vi "Read_Write_Temp_Cluster.vi"(3 "Template Info Array":T2[](array[typedef]) {"Tolerance" min=0.0 format="%#.4f"}, 4 "Mode":T1, 5 "Template File":path) -> (0 "Template Info Array Out":T2[](array[typedef]) {"Tolerance" min=0.0 format="%#.4f"})   [LabVIEW 2010]
uses:
  File_Template_Clus.ctl
  Controls/Global_mode.ctl
panel:
  # "> 20  or\n<20   or\n =20"
  # "<<Characters_to_Match>>  <<Replace_Whole_String_with_this>>"
  # "Channel_Name contains Characters to match or\nChannel_Name does not contain Characters to match"
  # "Channel_Name_A + Channel_Name_B or\nConcatenate Channel_Name_A and Channel_Name_B"
  # "> 20  or\n<20   or\n =20"
  # "<<Characters_to_Match>>  <<Replace_Whole_String_with_this>>"
  # "Channel_Name contains Characters to match or\nChannel_Name does not contain Characters to match"
  # "Channel_Name_A + Channel_Name_B or\nConcatenate Channel_Name_A and Channel_Name_B"
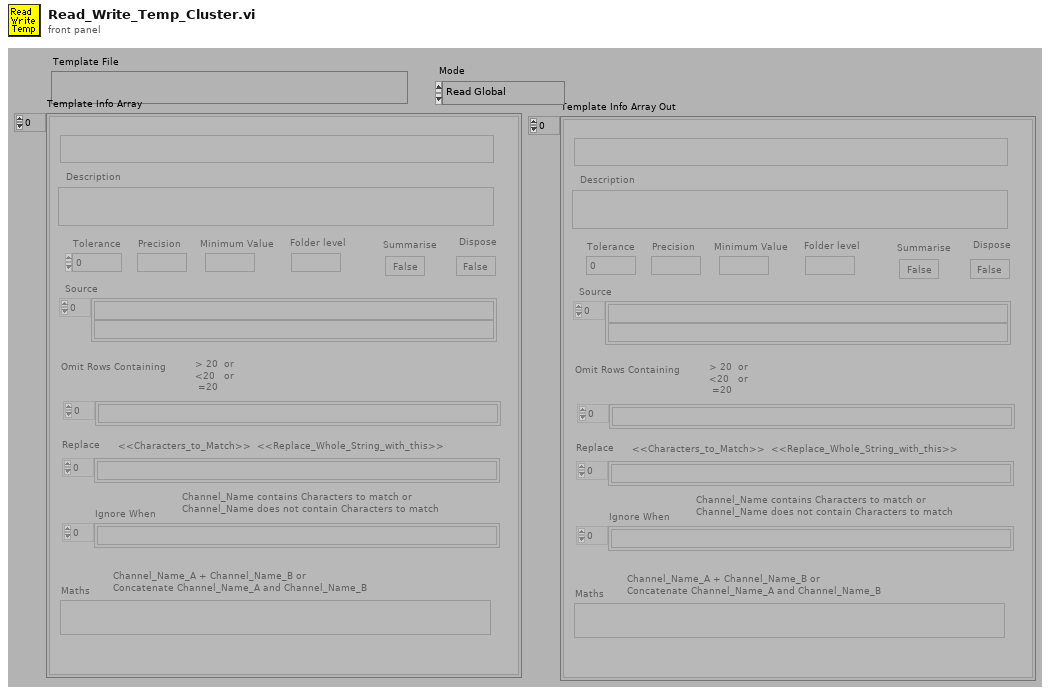
[diagram p1: front panel]
types:
  T1 = typedef "Global_mode.ctl" = enum16{"Read Global", "Load Global From File", "Write Global to File"}
  T2 = typedef "File_Template_Clus.ctl" = cluster{"Template Channel Name":string, "Description":string, "Tolerance":dbl, "Precision":string, "Folder level":string, "Source":string[], "Replace":string[], "Summarise":bool, "Dispose":bool, "Minimum Value":string, "Maths":string, "Omit Rows Containing":string[], "Ignore When":string[]}
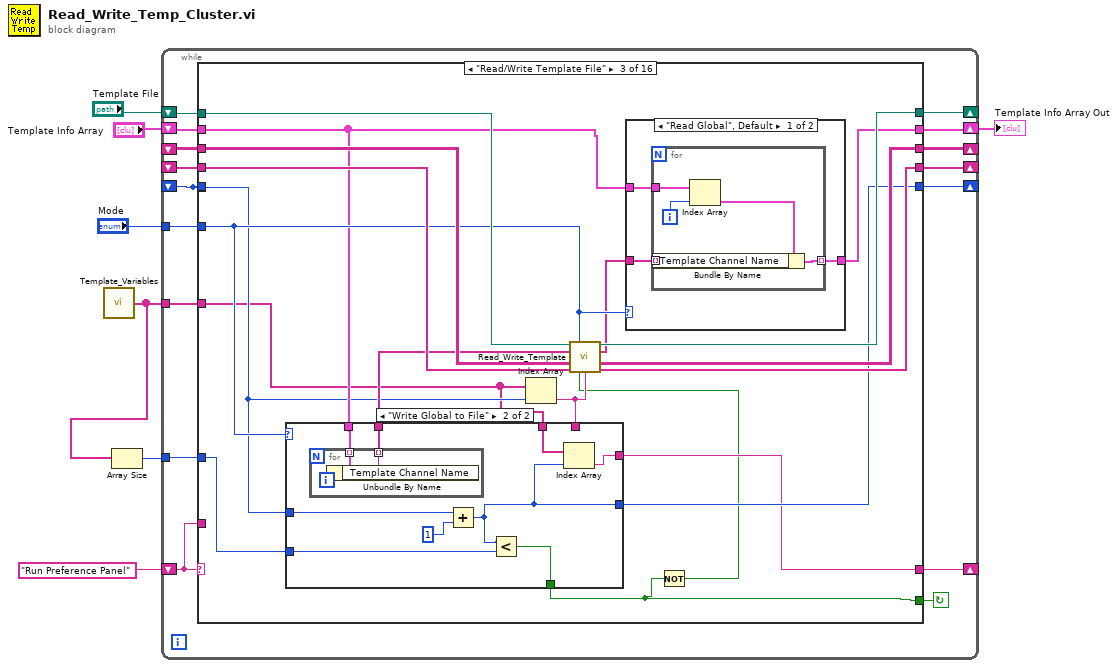
[diagram p0: block diagram]
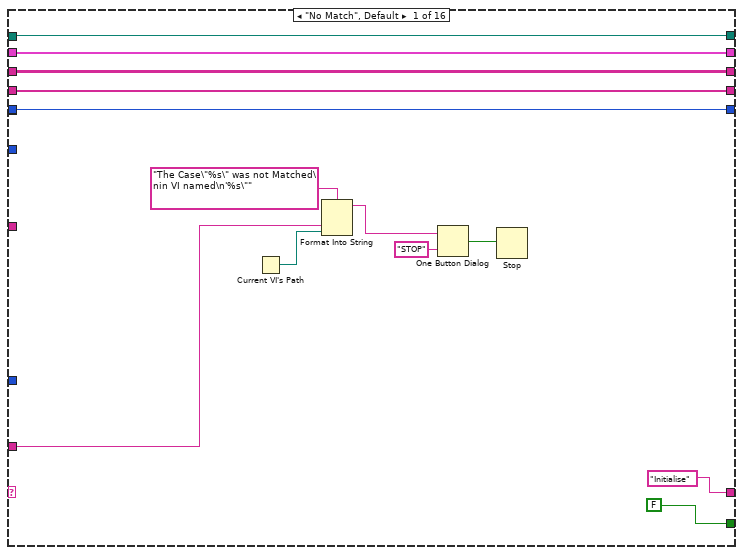
[diagram p2: hidden frame]
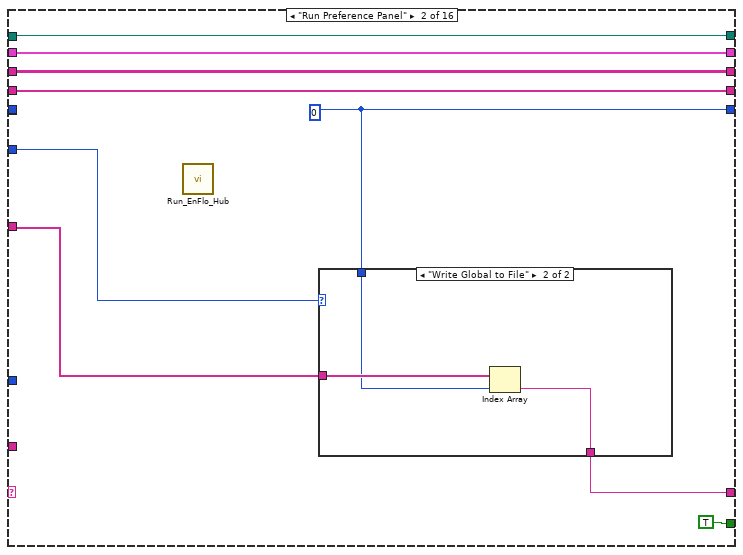
[diagram p3: hidden frame]
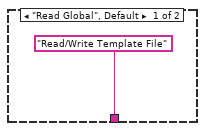
[diagram p4: hidden frame]
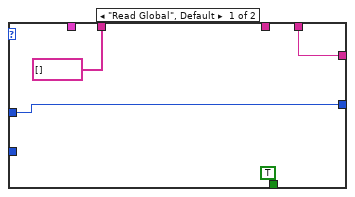
[diagram p6: hidden frame]
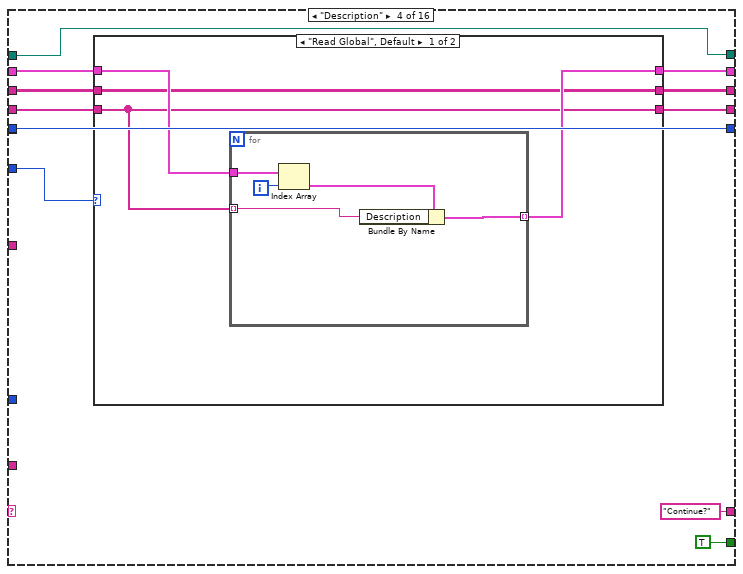
[diagram p7: hidden frame]
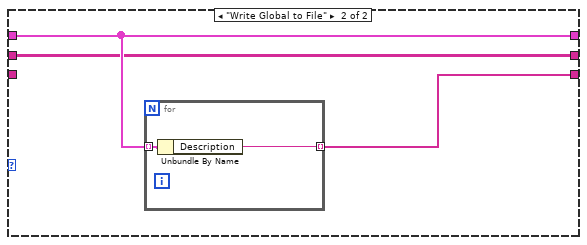
[diagram p8: hidden frame]
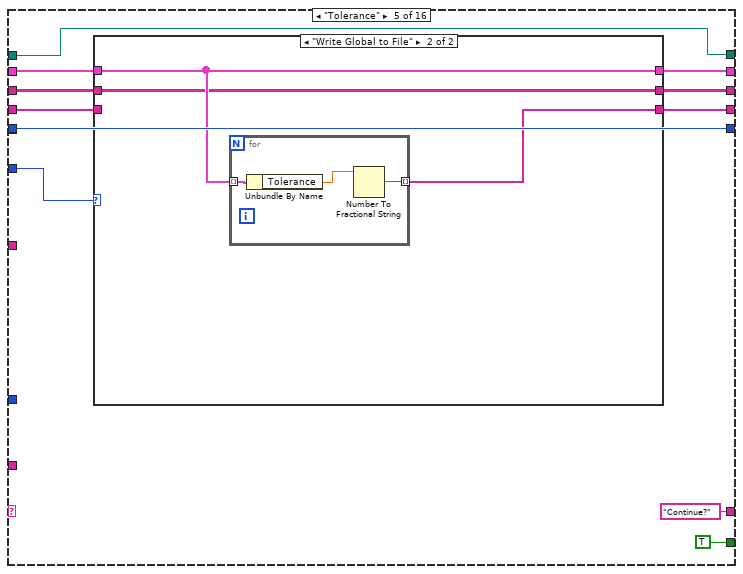
[diagram p9: hidden frame]
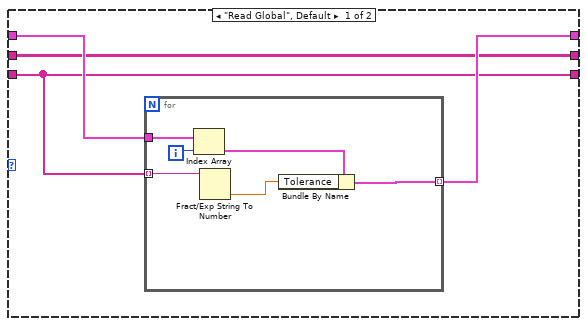
[diagram p10: hidden frame]
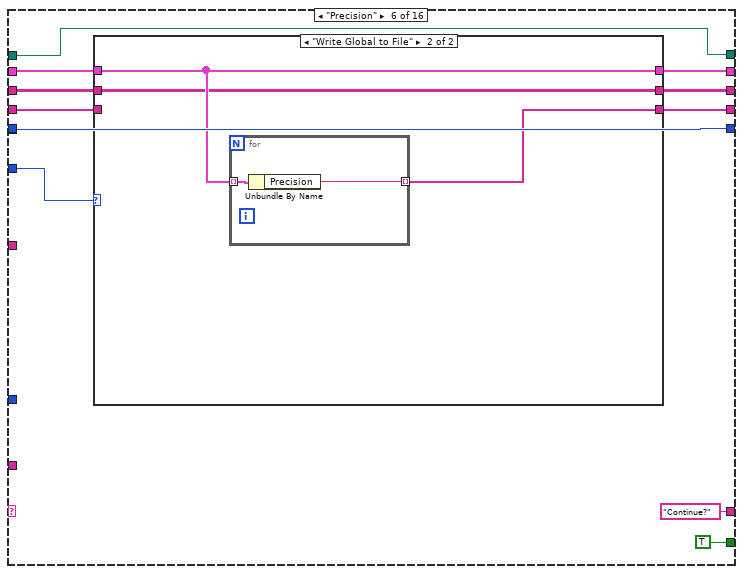
[diagram p11: hidden frame]
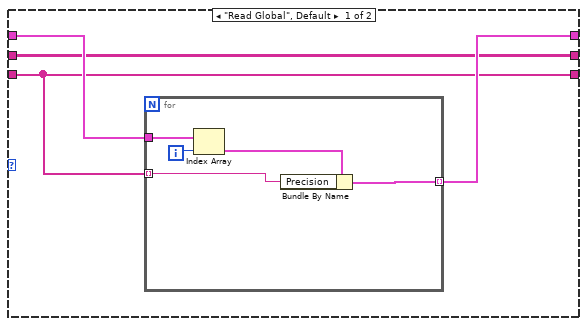
[diagram p12: hidden frame]
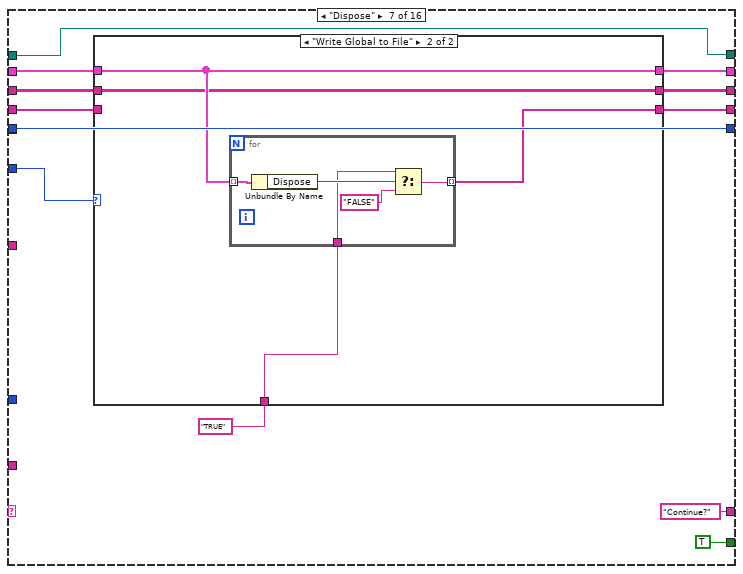
[diagram p13: hidden frame]
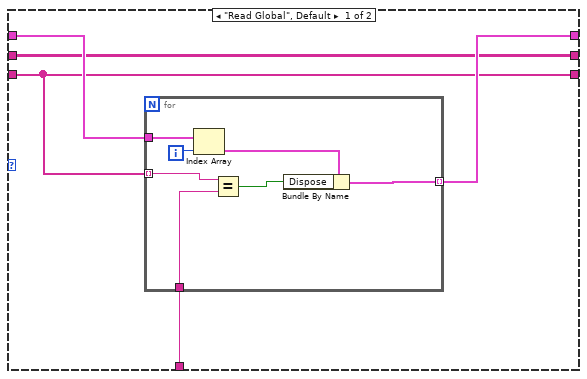
[diagram p14: hidden frame]
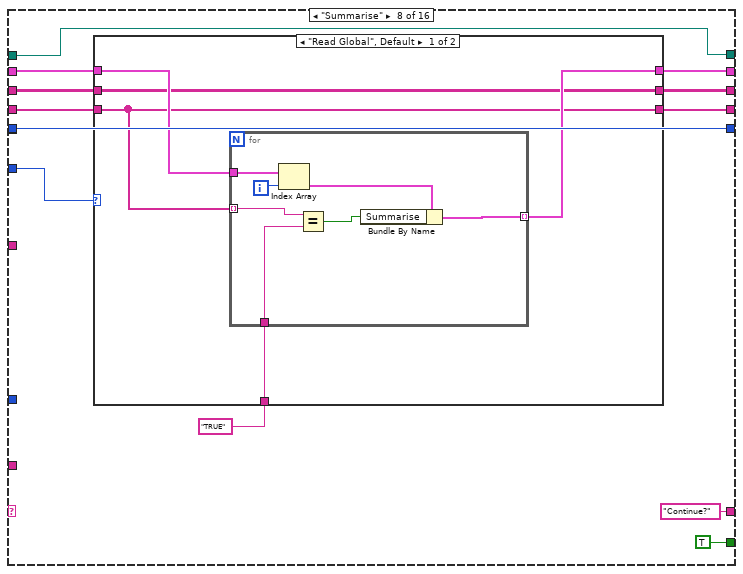
[diagram p15: hidden frame]
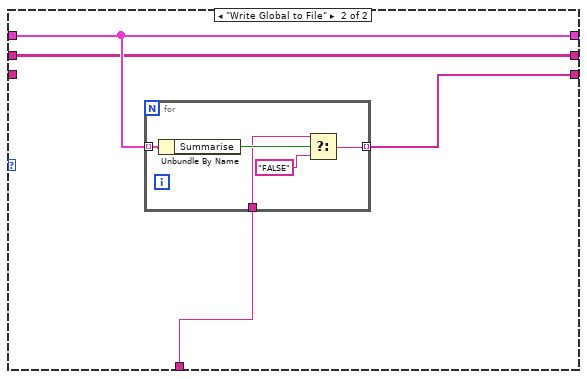
[diagram p16: hidden frame]
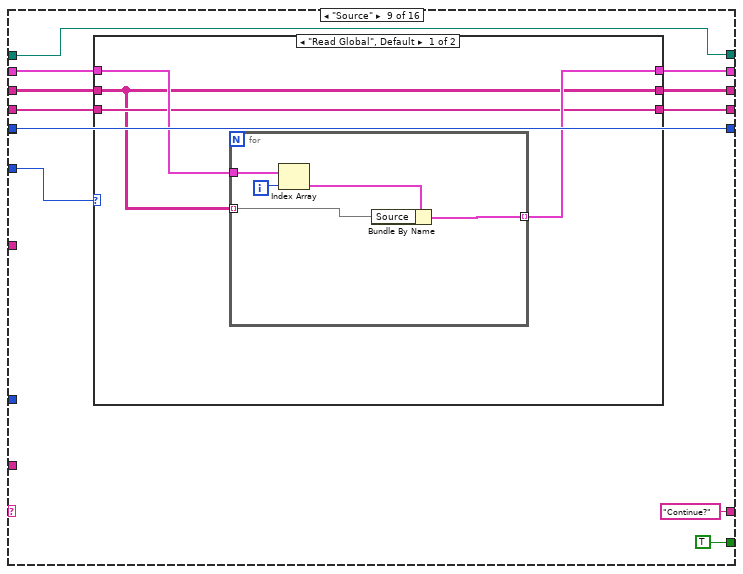
[diagram p17: hidden frame]
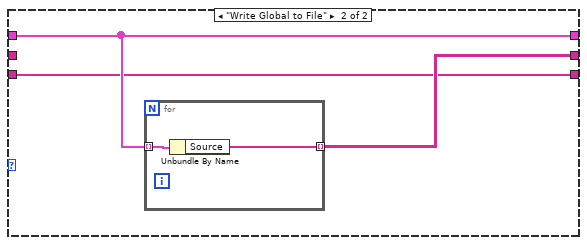
[diagram p18: hidden frame]
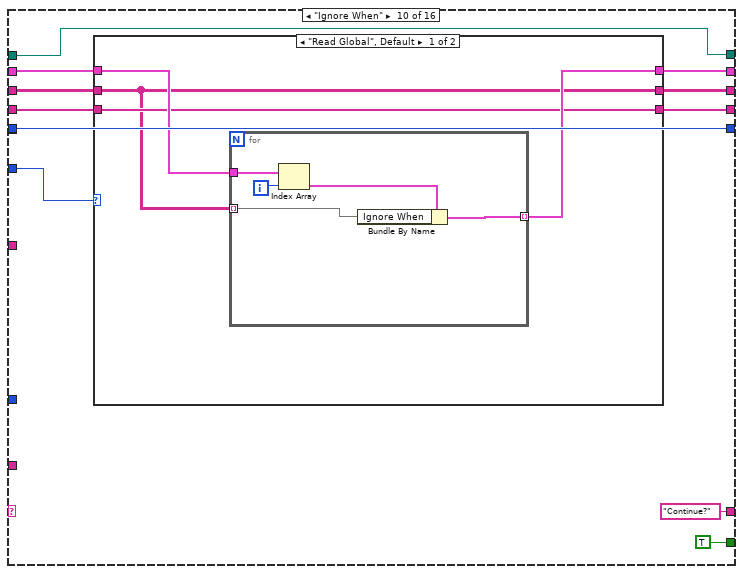
[diagram p19: hidden frame]
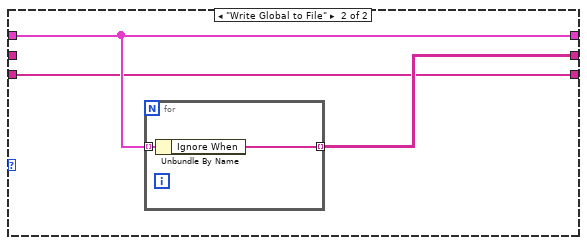
[diagram p20: hidden frame]
diagram:
  n1 = call "Template_Variables.vi"() -> ("Variable Names"=w1:string[])
  n2 = Array Size(array=w1) -> (size(s)=w2:i32)
  n3 = while {
    tunnel: w2 -> [w11]
    tunnel: "Mode" -> [w13]
    tunnel: w1 -> [w16]
    shift-left: "Template File" -> [w17]
    shift-right: [w8] -> _
    shift-left: _ -> [w10]
    shift-right: [w9] -> _
    shift-left: _ -> [w14]
    shift-right: [w18] -> _
    shift-left: _ -> [w15]
    shift-right: [w12] -> _
    shift-left: "Template Info Array" -> [w19]
    shift-right: [w20] -> w4
    shift-left: "Run Preference Panel" -> [w21]
    shift-right: [w22] -> _
    stop <- w23 continue-if-true
    n4 = case shown="\"Read/Write Template File\"" w21 {
      tunnel: [FALSE TRUE w51 TRUE TRUE TRUE TRUE TRUE TRUE TRUE TRUE TRUE TRUE TRUE TRUE w413] -> w23
      tunnel: ["Initialise" w39 w53 "Continue?" "Continue?" "Continue?" "Continue?" "Continue?" "Continue?" "Continue?" "Continue?" "Continue?" "Continue?" "Continue?" "Continue?" "Read/Write Template File"] -> w22
      tunnel: w21 -> [w31 _ _ _ _ _ _ _ _ _ _ _ _ _ _ _]
      tunnel: [w24 w43 w59 w95 w120 w147 w173 w206 w238 w263 w288 w313 w338 w363 w388 w419] -> w20
      tunnel: w19 -> [w24 w43 w58 w102 w127 w154 w180 w213 w245 w270 w295 w320 w345 w370 w395 w419]
      tunnel: [w27 w42 w68 w99 w124 w151 w177 w210 w242 w267 w292 w317 w342 w367 w392 w418] -> w12
      tunnel: [w26 w41 w67 w98 w123 w150 w176 w209 w241 w266 w291 w316 w341 w366 w391 w417] -> w18
      tunnel: [w28 w44 w65 w103 w128 w155 w181 w214 w246 w271 w296 w321 w346 w371 w396 w420] -> w8
      tunnel: w17 -> [w28 w44 w66 w103 w128 w155 w181 w214 w246 w271 w296 w321 w346 w371 w396 w420]
      tunnel: w10 -> [w25 _ w56 w93 w118 w145 w170 w203 w236 w261 w286 w311 w336 _ w386 w412]
      tunnel: w16 -> [_ w38 w54 _ _ _ _ _ _ _ _ _ _ _ _ w415]
      tunnel: w15 -> [w27 w42 w64 w100 w125 w152 w178 w211 w243 w268 w293 w318 w343 w368 w393 w418]
      tunnel: w14 -> [w26 w41 w63 w101 w126 w153 w179 w212 w244 w269 w294 w319 w344 w369 w394 w417]
      tunnel: w13 -> [_ w40 w60 w94 w119 w146 w171 w204 w237 w262 w287 w312 w337 w362 w387 w416]
      tunnel: w11 -> [_ _ w62 _ _ _ _ _ _ _ _ _ _ _ _ _]
      tunnel: w10 -> [_ _ _ _ _ _ _ _ _ _ _ _ _ w361 _ _]
      tunnel: [w25 w37 w55 w93 w118 w145 w170 w203 w236 w261 w286 w311 w336 w361 w386 w411] -> w9
      frame "No Match", Default {
        n5 = Current VI's Path() -> (path=w30:path)
        n6 = Format Into String(format string="The Case\"%s\" was not Matched\nin VI named\n'%s\"" ("Format String"), w31, w30) -> (resulting string=w34:string)  [unwired: 2 in, 1 out]
        n7 = One Button Dialog(message=w34, button name ("OK")="STOP") -> (true=w32:bool)
        n8 = Stop(stop? (T)=w32) -> ()
      }
      frame "Run Preference Panel" {
        w37 = 0
        n9 = call "Run_EnFlo_Hub.vi"() -> ()  [unwired: 8 out]
        n10 = case shown="\"Write Global to File\"" w40 {
          tunnel: ["Read/Write Template File" w48] -> w39
          tunnel: w38 -> [_ w49]
          tunnel: w37 -> [_ w47]
          frame "Read Global", Default {
          }
          frame "Write Global to File" {
            n11 = Index Array(array=w49, index=w47) -> (element=w48:string)
          }
        }
      }
      frame "Read/Write Template File" {
        n12 = Index Array(array=w54, index=w56) -> (element=w52:string)
        n13 = case shown="\"Write Global to File\"" w60 {
          tunnel: [w79 w84] -> w55
          tunnel: w56 -> [w79 w89]
          tunnel: w62 -> [_ w88]
          tunnel: [TRUE w87] -> w51
          tunnel: w58 -> [_ w86]
          tunnel: [string[] [] w85] -> w61
          tunnel: w54 -> [_ w83]
          tunnel: [w78 w82] -> w53
          tunnel: w52 -> [w78 _]
          frame "Read Global", Default {
          }
          frame "Write Global to File" {
            n14 = for {
              tunnel: w86 -> [w92] mode=indexing
              tunnel: [w91] -> w85 mode=indexing
              n15 = Unbundle By Name(w92) -> ("Template Channel Name"=w91:string)
            }
            n16 = Add(x=w89, y=1) -> (x+y=w84:i32)
            n17 = Less?(x=w84, y=w88) -> (x < y?=w87:bool)
            n18 = Index Array(array=w83, index=w84) -> (element=w82:string)
          }
        }
        n19 = Not(x=w51) -> (.not. x?=w50:bool)
        n20 = call "Read_Write_Template.vi"("Template File"=w66, "Mode"=w60, "Channel names In"=w61, "2D Info In"=w64, "1D Info In"=w63, "Save file"=w50, "Data type"=w52) -> ("Template File Out"=w65:path, "Template Ch Names Out"=w57:string[], "2D Info Out"=w68:string[][], "1D Info Out"=w67:string[])  [unwired: 1 in, 4 out]
        n21 = case shown="\"Read Global\", Default" w60 {
          tunnel: w58 -> [w71 w77]
          tunnel: [w70 w77] -> w59
          tunnel: w57 -> [w69 _]
          frame "Read Global", Default {
            n22 = for {
              tunnel: w71 -> [w74]
              tunnel: [w76] -> w70 mode=indexing
              tunnel: w69 -> [w75] mode=indexing
              i -> [w73]
              n23 = Index Array(array=w74, index=w73) -> (element=w72:T2)
              n24 = Bundle By Name(cluster=w72, "Template Channel Name"=w75) -> (w76:T2)
            }
          }
          frame "Write Global to File" {
          }
        }
      }
      frame "Description" {
        n25 = case shown="\"Read Global\", Default" w94 {
          tunnel: w102 -> [w107 w115]
          tunnel: w101 -> [w104 _]
          tunnel: [w106 w115] -> w95
          tunnel: w100 -> [w105 w113]
          tunnel: [w105 w113] -> w99
          tunnel: [w104 w114] -> w98
          frame "Read Global", Default {
            n26 = for {
              tunnel: w107 -> [w111]
              tunnel: w104 -> [w108] mode=indexing
              tunnel: [w109] -> w106 mode=indexing
              i -> [w112]
              n27 = Index Array(array=w111, index=w112) -> (element=w110:T2)
              n28 = Bundle By Name(cluster=w110, "Description"=w108) -> (w109:T2)
            }
          }
          frame "Write Global to File" {
            n29 = for {
              tunnel: w115 -> [w117] mode=indexing
              tunnel: [w116] -> w114 mode=indexing
              n30 = Unbundle By Name(w117) -> ("Description"=w116:string)
            }
          }
        }
      }
      frame "Tolerance" {
        n31 = case shown="\"Write Global to File\"" w119 {
          tunnel: w127 -> [w132 w141]
          tunnel: w126 -> [w129 _]
          tunnel: [w131 w141] -> w120
          tunnel: w125 -> [w130 w139]
          tunnel: [w130 w139] -> w124
          tunnel: [w129 w140] -> w123
          frame "Read Global", Default {
            n32 = for {
              tunnel: w132 -> [w137]
              tunnel: w129 -> [w135] mode=indexing
              tunnel: [w133] -> w131 mode=indexing
              i -> [w138]
              n33 = Index Array(array=w137, index=w138) -> (element=w136:T2)
              n34 = Fract/Exp String To Number(string=w135) -> (number=w134:dbl)  [unwired: 4 out]
              n35 = Bundle By Name(cluster=w136, "Tolerance"=w134) -> (w133:T2)
            }
          }
          frame "Write Global to File" {
            n36 = for {
              tunnel: w141 -> [w144] mode=indexing
              tunnel: [w142] -> w140 mode=indexing
              n37 = Unbundle By Name(w144) -> ("Tolerance"=w143:dbl)
              n38 = Number To Fractional String(number=w143) -> (F-format string=w142:string)  [unwired: 3 out]
            }
          }
        }
      }
      frame "Precision" {
        n39 = case shown="\"Write Global to File\"" w146 {
          tunnel: w154 -> [w159 w167]
          tunnel: w153 -> [w156 _]
          tunnel: [w158 w167] -> w147
          tunnel: w152 -> [w157 w165]
          tunnel: [w157 w165] -> w151
          tunnel: [w156 w166] -> w150
          frame "Read Global", Default {
            n40 = for {
              tunnel: w159 -> [w163]
              tunnel: w156 -> [w160] mode=indexing
              tunnel: [w161] -> w158 mode=indexing
              i -> [w164]
              n41 = Index Array(array=w163, index=w164) -> (element=w162:T2)
              n42 = Bundle By Name(cluster=w162, "Precision"=w160) -> (w161:T2)
            }
          }
          frame "Write Global to File" {
            n43 = for {
              tunnel: w167 -> [w169] mode=indexing
              tunnel: [w168] -> w166 mode=indexing
              n44 = Unbundle By Name(w169) -> ("Precision"=w168:string)
            }
          }
        }
      }
      frame "Dispose" {
        n45 = case shown="\"Write Global to File\"" w171 {
          tunnel: w180 -> [w186 w197]
          tunnel: w179 -> [w183 _]
          tunnel: [w185 w197] -> w173
          tunnel: w178 -> [w184 w195]
          tunnel: [w184 w195] -> w177
          tunnel: [w183 w196] -> w176
          tunnel: "TRUE" ("y") -> [w182 w194]
          frame "Read Global", Default {
            n46 = for {
              tunnel: w186 -> [w192]
              tunnel: w183 -> [w189] mode=indexing
              tunnel: [w190] -> w185 mode=indexing
              tunnel: w182 -> [w187]
              i -> [w193]
              n47 = Index Array(array=w192, index=w193) -> (element=w191:T2)
              n48 = Equal?(x=w189, y=w187) -> (x = y?=w188:bool)
              n49 = Bundle By Name(cluster=w191, "Dispose"=w188) -> (w190:T2)
            }
          }
          frame "Write Global to File" {
            n50 = for {
              tunnel: w197 -> [w202] mode=indexing
              tunnel: [w198] -> w196 mode=indexing
              tunnel: w194 -> [w200]
              n51 = Unbundle By Name(w202) -> ("Dispose"=w201:bool)
              n52 = Select(t=w200, s=w201, f="FALSE") -> (s? t:f=w198:string)
            }
          }
        }
      }
      frame "Summarise" {
        n53 = case shown="\"Read Global\", Default" w204 {
          tunnel: w213 -> [w219 w230]
          tunnel: w212 -> [w216 _]
          tunnel: [w218 w230] -> w206
          tunnel: w211 -> [w217 w228]
          tunnel: [w217 w228] -> w210
          tunnel: [w216 w229] -> w209
          tunnel: "TRUE" ("y") -> [w215 w227]
          frame "Read Global", Default {
            n54 = for {
              tunnel: w219 -> [w225]
              tunnel: w216 -> [w222] mode=indexing
              tunnel: [w223] -> w218 mode=indexing
              tunnel: w215 -> [w220]
              i -> [w226]
              n55 = Index Array(array=w225, index=w226) -> (element=w224:T2)
              n56 = Equal?(x=w222, y=w220) -> (x = y?=w221:bool)
              n57 = Bundle By Name(cluster=w224, "Summarise"=w221) -> (w223:T2)
            }
          }
          frame "Write Global to File" {
            n58 = for {
              tunnel: w230 -> [w235] mode=indexing
              tunnel: [w231] -> w229 mode=indexing
              tunnel: w227 -> [w233]
              n59 = Unbundle By Name(w235) -> ("Summarise"=w234:bool)
              n60 = Select(t=w233, s=w234, f="FALSE") -> (s? t:f=w231:string)
            }
          }
        }
      }
      frame "Source" {
        n61 = case shown="\"Read Global\", Default" w237 {
          tunnel: w245 -> [w250 w258]
          tunnel: w244 -> [w248 w256]
          tunnel: [w249 w258] -> w238
          tunnel: w243 -> [w247 _]
          tunnel: [w247 w257] -> w242
          tunnel: [w248 w256] -> w241
          frame "Read Global", Default {
            n62 = for {
              tunnel: w250 -> [w254]
              tunnel: w247 -> [w251] mode=indexing
              tunnel: [w252] -> w249 mode=indexing
              i -> [w255]
              n63 = Index Array(array=w254, index=w255) -> (element=w253:T2)
              n64 = Bundle By Name(cluster=w253, "Source"=w251) -> (w252:T2)
            }
          }
          frame "Write Global to File" {
            n65 = for {
              tunnel: w258 -> [w260] mode=indexing
              tunnel: [w259] -> w257 mode=indexing
              n66 = Unbundle By Name(w260) -> ("Source"=w259:string[])
            }
          }
        }
      }
      frame "Ignore When" {
        n67 = case shown="\"Read Global\", Default" w262 {
          tunnel: w270 -> [w275 w283]
          tunnel: w269 -> [w273 w281]
          tunnel: [w274 w283] -> w263
          tunnel: w268 -> [w272 _]
          tunnel: [w272 w282] -> w267
          tunnel: [w273 w281] -> w266
          frame "Read Global", Default {
            n68 = for {
              tunnel: w275 -> [w279]
              tunnel: w272 -> [w276] mode=indexing
              tunnel: [w277] -> w274 mode=indexing
              i -> [w280]
              n69 = Index Array(array=w279, index=w280) -> (element=w278:T2)
              n70 = Bundle By Name(cluster=w278, "Ignore When"=w276) -> (w277:T2)
            }
          }
          frame "Write Global to File" {
            n71 = for {
              tunnel: w283 -> [w285] mode=indexing
              tunnel: [w284] -> w282 mode=indexing
              n72 = Unbundle By Name(w285) -> ("Ignore When"=w284:string[])
            }
          }
        }
      }
      frame "Replace" {
        n73 = case shown="\"Read Global\", Default" w287 {
          tunnel: w295 -> [w300 w308]
          tunnel: w294 -> [w298 w306]
          tunnel: [w299 w308] -> w288
          tunnel: w293 -> [w297 _]
          tunnel: [w297 w307] -> w292
          tunnel: [w298 w306] -> w291
          frame "Read Global", Default {
            n74 = for {
              tunnel: w300 -> [w304]
              tunnel: w297 -> [w301] mode=indexing
              tunnel: [w302] -> w299 mode=indexing
              i -> [w305]
              n75 = Index Array(array=w304, index=w305) -> (element=w303:T2)
              n76 = Bundle By Name(cluster=w303, "Replace"=w301) -> (w302:T2)
            }
          }
          frame "Write Global to File" {
            n77 = for {
              tunnel: w308 -> [w310] mode=indexing
              tunnel: [w309] -> w307 mode=indexing
              n78 = Unbundle By Name(w310) -> ("Replace"=w309:string[])
            }
          }
        }
      }
      frame "Maths" {
        n79 = case shown="\"Read Global\", Default" w312 {
          tunnel: w320 -> [w325 w333]
          tunnel: w319 -> [w322 _]
          tunnel: [w324 w333] -> w313
          tunnel: w318 -> [w323 w331]
          tunnel: [w323 w331] -> w317
          tunnel: [w322 w332] -> w316
          frame "Read Global", Default {
            n80 = for {
              tunnel: w325 -> [w329]
              tunnel: w322 -> [w326] mode=indexing
              tunnel: [w327] -> w324 mode=indexing
              i -> [w330]
              n81 = Index Array(array=w329, index=w330) -> (element=w328:T2)
              n82 = Bundle By Name(cluster=w328, "Maths"=w326) -> (w327:T2)
            }
          }
          frame "Write Global to File" {
            n83 = for {
              tunnel: w333 -> [w335] mode=indexing
              tunnel: [w334] -> w332 mode=indexing
              n84 = Unbundle By Name(w335) -> ("Maths"=w334:string)
            }
          }
        }
      }
      frame "Omit" {
        n85 = case shown="\"Write Global to File\"" w337 {
          tunnel: w345 -> [w350 w358]
          tunnel: w344 -> [w348 w356]
          tunnel: [w349 w358] -> w338
          tunnel: w343 -> [w347 _]
          tunnel: [w347 w357] -> w342
          tunnel: [w348 w356] -> w341
          frame "Read Global", Default {
            n86 = for {
              tunnel: w350 -> [w354]
              tunnel: w347 -> [w351] mode=indexing
              tunnel: [w352] -> w349 mode=indexing
              i -> [w355]
              n87 = Index Array(array=w354, index=w355) -> (element=w353:T2)
              n88 = Bundle By Name(cluster=w353, "Omit Rows Containing"=w351) -> (w352:T2)
            }
          }
          frame "Write Global to File" {
            n89 = for {
              tunnel: w358 -> [w360] mode=indexing
              tunnel: [w359] -> w357 mode=indexing
              n90 = Unbundle By Name(w360) -> ("Omit Rows Containing"=w359:string[])
            }
          }
        }
      }
      frame "Folder level" {
        n91 = case shown="\"Write Global to File\"" w362 {
          tunnel: w370 -> [w375 w383]
          tunnel: w369 -> [w372 _]
          tunnel: [w374 w383] -> w363
          tunnel: w368 -> [w373 w381]
          tunnel: [w373 w381] -> w367
          tunnel: [w372 w382] -> w366
          frame "Read Global", Default {
            n92 = for {
              tunnel: w375 -> [w379]
              tunnel: w372 -> [w376] mode=indexing
              tunnel: [w377] -> w374 mode=indexing
              i -> [w380]
              n93 = Index Array(array=w379, index=w380) -> (element=w378:T2)
              n94 = Bundle By Name(cluster=w378, "Folder level"=w376) -> (w377:T2)
            }
          }
          frame "Write Global to File" {
            n95 = for {
              tunnel: w383 -> [w385] mode=indexing
              tunnel: [w384] -> w382 mode=indexing
              n96 = Unbundle By Name(w385) -> ("Folder level"=w384:string)
            }
          }
        }
      }
      frame "Minimum Value" {
        n97 = case shown="\"Write Global to File\"" w387 {
          tunnel: w395 -> [w400 w408]
          tunnel: w394 -> [w397 _]
          tunnel: [w399 w408] -> w388
          tunnel: w393 -> [w398 w406]
          tunnel: [w398 w406] -> w392
          tunnel: [w397 w407] -> w391
          frame "Read Global", Default {
            n98 = for {
              tunnel: w400 -> [w404]
              tunnel: w397 -> [w402] mode=indexing
              tunnel: [w401] -> w399 mode=indexing
              i -> [w405]
              n99 = Index Array(array=w404, index=w405) -> (element=w403:T2)
              n100 = Bundle By Name(cluster=w403, "Minimum Value"=w402) -> (w401:T2)
            }
          }
          frame "Write Global to File" {
            n101 = for {
              tunnel: w408 -> [w410] mode=indexing
              tunnel: [w409] -> w407 mode=indexing
              n102 = Unbundle By Name(w410) -> ("Minimum Value"=w409:string)
            }
          }
        }
      }
      frame "Continue?" {
        n103 = Array Size(array=w415) -> (size(s)=w414:i32)
        n104 = case shown="\"Read Global\", Default" w416 {
          tunnel: w414 -> [w426 _]
          tunnel: [w425 TRUE] -> w413
          tunnel: w412 -> [w423 w427]
          tunnel: [w422 w427] -> w411
          frame "Read Global", Default {
            n105 = Add(x=w423, y=1) -> (x+y=w422:i32)
            n106 = Less?(x=w422, y=w426) -> (x < y?=w425:bool)
          }
          frame "Write Global to File" {
          }
        }
      }
    }
  }
  "Template Info Array Out" <- w4
